vi "Register JSON.vi"(7 "Options":string="{}", 8 "Error in":errorcluster, 9 "Time out (1000 ms)":i32=1000, 10 "Procedure URI":string, 11 "WAMP Client in":refnum<class "WAMP Client.lvclass">) -> (0 "Error out":errorcluster, 3 "WAMP Client out":refnum<class "WAMP Client.lvclass">, 5 "WAMP Error":T1={"Error URI"="", "Error Arguments"="", "Error ArgumentKw"="{}", "Error Details"="{}", "Associated LabVIEW Error"={"status"=FALSE, "code"=0, "source"=""}})   [LabVIEW 2020, in "wamplv.lvlib" / "WAMP Client.lvclass"]
uses:
  WAMP Client.lvclass
  TypeDefs/Error or abort detail (JSON).ctl
  WAMP Client.lvclass/WAMP Client.ctl
  1e58c327-2179-4469-bfa1-996a18af625e.vi
  <vilib>/Utility/error.llb/Error Cluster From Error Code.vi
  wamplv.lvlib
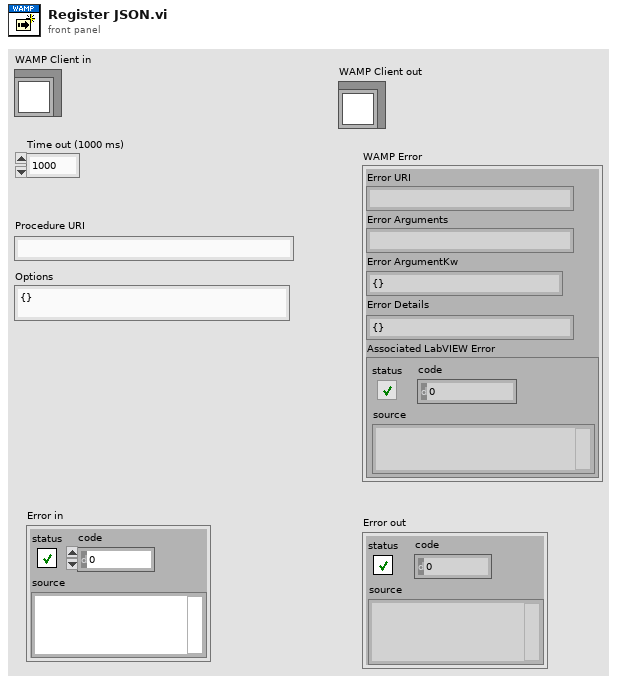
[diagram p1: front panel]
types:
  T1 = typedef "wamplv.lvlib/Error or abort detail (JSON).ctl" = cluster{"Error URI":string, "Error Arguments":string, "Error ArgumentKw":string, "Error Details":string, "Associated LabVIEW Error":errorcluster}
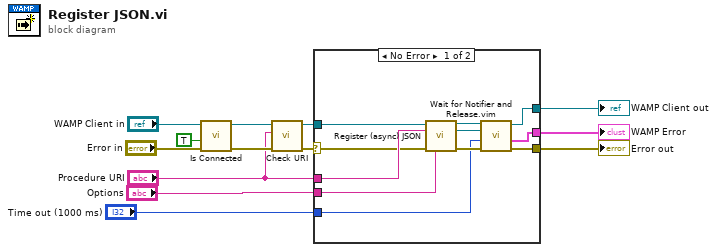
[diagram p0: block diagram]
diagram:
  n1 = call "Is Connected.vi"("error in"="Error in", "Raise error if not connected"=TRUE, "WAMP Client in"="WAMP Client in") -> ("error out"=w5:errorcluster, "WAMP Client out"=w3:refnum<class "WAMP Client.lvclass">)  [unwired: 6 in, 1 out]
  n2 = call "Check URI.vi"("error in (no error)"=w5, "URI"="Procedure URI", "WAMP Client in"=w3) -> ("error out"=w4:errorcluster, "WAMP Client out"=w2:refnum<class "WAMP Client.lvclass">)  [unwired: 5 in, 2 out]
  n3 = case shown="No Error" w4 {
    selector: w4 -> [w17 w26]
    tunnel: [w19 w26] -> w10
    tunnel: [w15 w25] -> w13
    tunnel: w2 -> [w22 w25]
    tunnel: "Procedure URI" -> [w24 _]
    tunnel: "Options" -> [w23 _]
    tunnel: "Time out (1000 ms)" -> [w20 _]
    tunnel: [w18 _] -> w9
    frame No Error {
      n4 = call-dynamic "Register (async) JSON.vi"("WAMP Client in"=w22, "Options"=w23, "Procedure URI"=w24, "error in (no error)"=w17) -> ("WAMP Client out"=w16:refnum<class "WAMP Client.lvclass">, "notifier out"=w14:refnum<notifier>, "error out"=w21:errorcluster)  [unwired: 9 in]
      n5 = call "Wait for Notifier and Release.vim"("error in (no error)"=w21, "timeout in ms (0)"=w20, "Notifier in"=w14, "WAMP Client in"=w16) -> ("error out"=w19:errorcluster, "WAMP Error"=w18:T1, "WAMP Client out"=w15:refnum<class "WAMP Client.lvclass">)  [unwired: 4 in, 1 out]
    }
    frame Error {
    }
  }
  "Error out" <- w10
  "WAMP Client out" <- w13
  "WAMP Error" <- w9
